vi "robotGoToBehindTheBall.vi"(6 "AttackingOurselves":bool=TRUE, 8 "error in (no error)":errorcluster, 9 "BallRef":refnum<class "Ball.lvclass">, 10 "Robot":refnum<class "Robot.lvclass">, 11 "Utilities in":refnum<class "Utilities.lvclass">) -> (0 "error out":errorcluster, 1 "dest_y":dbl, 2 "dest_x":dbl, 3 "Utilities out":refnum<class "Utilities.lvclass">)   [LabVIEW 2020, in "Utilities.lvclass"]
uses:
  Utilities.lvclass
  Ball_class/Ball.lvclass
  Robot_class/Robot.lvclass
  KickToSkill_class/KickToSkill.lvclass
  Object_class/Object.lvclass/Object.ctl
  <vilib>/Analysis/baseanly.llb/Unit Vector (DBL).vi
  Object_class/Read x.vi
  Object_class/Read y.vi
  <vilib>/Analysis/NI_AALBase.lvlib
panel:
  out "KickToSkill out":refnum<class "KickToSkill.lvclass">
  in  "KickToSkill in":refnum<class "KickToSkill.lvclass">
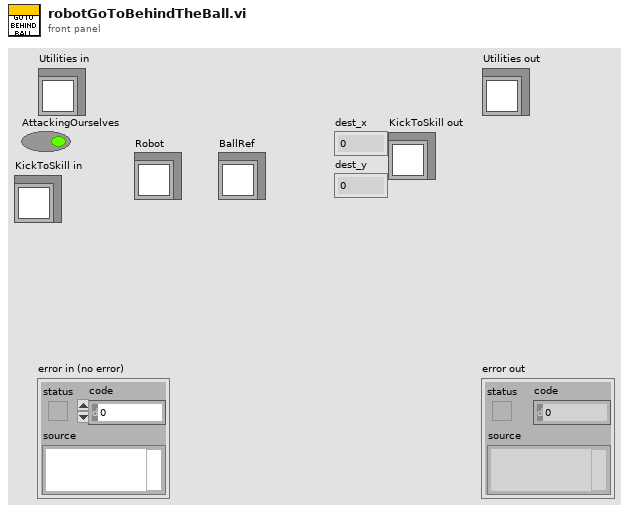
[diagram p1: front panel]
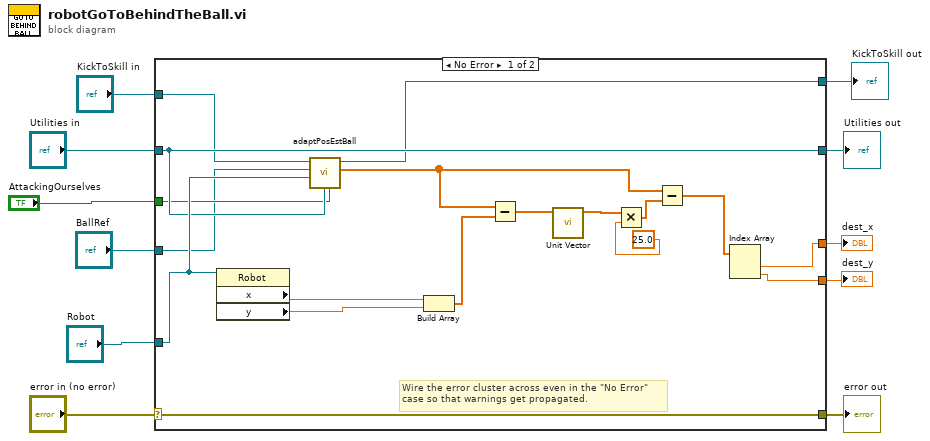
[diagram p0: block diagram]
diagram:
  n1 = case shown="No Error" "error in (no error)" {
    selector: "error in (no error)" -> [w29 w31]
    tunnel: [w29 w31] -> w10
    tunnel: [w16 w30] -> w8
    tunnel: "Utilities in" -> [w16 w30]
    tunnel: "BallRef" -> [w14 _]
    tunnel: "Robot" -> [w17 _]
    tunnel: [w20 _] -> w5
    tunnel: [w19 _] -> w4
    tunnel: "AttackingOurselves" -> [w15 _]
    tunnel: "KickToSkill in" -> [w13 _]
    tunnel: [w12 _] -> w1
    frame No Error {
      # "Wire the error cluster across even in the \"No Error\"\ncase so that warnings get propagated."
      n2 = property class="Robot"(reference=w17) -> ("x"=w28:dbl, "y"=w27:dbl)  [unwired: 1 in, 2 out]
      n3 = call "adaptPosEstBall.vi"("AttakingOurselves"=w15, "Utilities.lvclass"=w16, "Robot"=w17, "BallRef"=w14, "KickToSkill in"=w13) -> ("Pos_est adapted"=w18:dbl[], "KickToSkill out"=w12:refnum<class "KickToSkill.lvclass">)  [unwired: 4 in, 1 out]
      n4 = Build Array(w28, w27) -> (w26:dbl[])
      n5 = Subtract(x=w18, y=w26) -> (x-y=w25:dbl[])
      n6 = call-poly <vilib>:"Unit Vector.vi"("Input Vector"=w25) -> ("Unit Vector"=w23:dbl[])  [unwired: 8 in, 2 out]
      n7 = Multiply(x=w23, y=25.0) -> (x*y=w22:dbl[])
      n8 = Subtract(x=w18, y=w22) -> (x-y=w21:dbl[])
      n9 = Index Array(array=w21) -> (element #1=w20:dbl, element #2=w19:dbl)  [unwired: 2 in]
    }
    frame Error {
    }
  }
  "error out" <- w10
  "Utilities out" <- w8
  "dest_x" <- w5
  "dest_y" <- w4
  "KickToSkill out" <- w1
